vi "Dashboard Main.vi"() -> ()   [LabVIEW 2013]
uses:
  Vision Stuff/TargetType.ctl
  <vilib>/event_ctls.llb/eventvkey.ctl
  <vilib>/Rock Robotics/WPI/Dashboard/WPI_DashboardLogging Global.vi
  <vilib>/Utility/config.llb/Write Key (String).vi
  <vilib>/Utility/config.llb/Write Key (I32).vi
  <vilib>/Utility/config.llb/NI_LVConfig.lvlib
panel:
  out "Image Message":string="Timeout in Camera Communications"
  in  "Rec Mode":enum32{"Stop", "Record", "Playback"}(radio)
  in  "Dashboard Tab":T1(tab)
  in  "PID rotation":bool
  in  "Use Gyro":bool=TRUE
  in  "Camera Settings":T2={"Frame Rate"=30, "Compression"=30, "Size"=1} {"Frame Rate" scale=1.0..30.0; "Size" items=["640x480", "320x240", "160x120"]}
  out "MotorSliders R":cluster{"MotorSlide1":dbl, "MotorSlide2":dbl} {"MotorSlide2" scale=-1.0..1.0 scale format="%#_2e"; "MotorSlide1" scale=-1.0..1.0 scale format="%#_2e"}
  out "MotorChart R":cluster{"Numeric":dbl, "Numeric":dbl}(graph)
  out "MotorSliders L":T3 {"MotorSlide4 2" scale=0.0..14.0 scale format="%#_2e"; "MotorSlide2" scale=-1.0..1.0 scale format="%#_2e"; "MotorSlide1" scale=-1.0..1.0 scale format="%#_2e"}
  out "MotorChart L":T4(graph)
  out "JS1 Z":dbl(slide) scale=-1.0..1.0 scale format="%#_2e"
  out "Joystick 1":cluster{"X":dbl, "Y":dbl}[](graph)
  out "JS Buttons 1":T5
  out "JS2 Z":dbl(slide) scale=-1.0..1.0 scale format="%#_2e"
  out "Joystick 2":cluster{"X":dbl, "Y":dbl}[](graph)
  out "JS Buttons 2":T5
  out "Mode":T6(ring)=enum."Auto Disabled"
  out "Camera IP":string
  in  "DB Camera Config":bool
  out "fps":dbl format="%#.1g"
  out "Mbps":dbl format="%#.1g"
  out "Mbps 2":bool
  out "LED 1":bool
  in  "Op joystick select":string(combo)="Regular"
  in  "Driver joystick select":string(combo)="Regular"
  in  "Automatic reload?":bool
  out "Ultrasonic":dbl
  in  "Joystick":dbl=4.2
  in  "Gain":dbl=0.03
  out "Angle":dbl(knob) scale=0.0..360.0
  out "Hardstop position":bool
  out "Hardstop RPM":dbl
  out "Hardstop Encoder Distance":dbl
  in  "Slider 1":dbl(slide) scale=0.0..100.0
  in  "Value":dbl
  in  "Var#":dbl
  in  "Auton#":dbl
  in  "Update":bool
  in  "Auton's":string(combo)="OneBall"
  in  "Checkbox 2":bool
  in  "Checkbox 1":bool
  in  "Test Slider":dbl(slide) scale=0.0..100.0 scale format="%#_3g"
  in  "On/Off":bool caption="Solenoid"
  in  "Test Name":u16(ring) items=["Select the test to run...", "Example Test", "-------------------------------", "List of tests is built in robot code.", "Replace with your own automated tests."]
  in  "Test Tree":string(tree)
  in  "Motor":cluster{"Value":dbl, "Enable":bool} {"Value" scale=-1.0..1.0 scale format="%#_3g"}
  out "Progress":T7 {"Test Progress" scale=0.0..100.0}
  in  "Rev/Fwd":cluster{"Forward":bool, "Reverse":bool}
  in  "Test Ring":u16(ring) items=["Auto", "Fixed indoor", "Fixed outdoor 1", "Fixed outdoor 2", "Fixed fluorescent 1", "Fixed fluorescent 2", "Hold current"]
  in  "Listbox":i32(listbox)
  out "Tree":string(tree)
  out "Scores.State":T8
  out "Distance (ft)":dbl
  out "Heatmap":T9(plugin-control)
  out "Camera Image 2":T9(plugin-control)
  out "Ball X-Axis":sgl
  out "Camera Image":T9(plugin-control)
  in  "Enable":bool=TRUE
  # "ON"
  # "ON"
  # "OFF"
  # "Left"
  # "Front"
  # "Right"
  # "OFF"
  # "ON"
  # "Battery"
  # "OFF"
  # "Customize by placing controls and indicators here and name to\nmatch Dashboard Variables on robot."
  # "This tab is a great place for autonomous settings and validation.\nCustomize by placing controls and indicators here and name to\nmatch Dashboard Variables on robot."
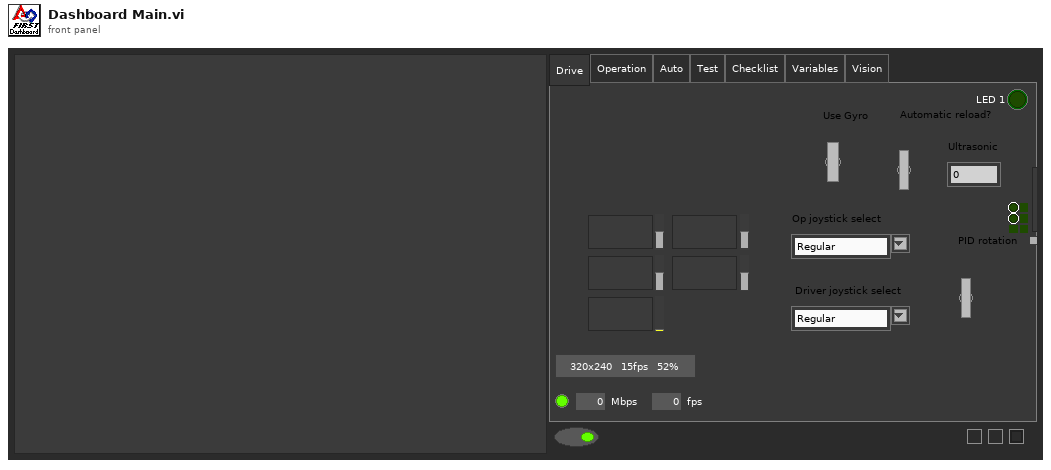
[diagram p1: front panel]
types:
  T1 = enum32{"Drive", "Operation", "Auto", "Test", "Checklist", "Variables", "Vision"}
  T2 = cluster{"Frame Rate":i32, "Compression":i32, "Size":u16}
  T3 = cluster{"MotorSlide1":dbl, "MotorSlide2":dbl, "MotorSlide4 2":dbl}
  T4 = cluster{"Numeric":dbl, "Numeric":dbl, "Battery":sgl}
  T5 = cluster{bool, bool, bool, bool, bool, bool, bool, bool, bool, bool, bool, bool}
  T6 = enum8{"Tele-Op Disabled", "Tele-Op Enabled", "Auto Disabled", "Auto Enabled", "Test Disabled", "Test Enabled", ""}
  T7 = cluster{"Test Progress":u8, "Test Progress Text":string}
  T8 = typedef "TargetType.ctl" = enum16{"Not Hot", "Hot"}
  T9 = typedef "IMAQ Image.ctl" = refnum<image>
  T10 = typedef "Image Type" = u32
  T11 = enum32{"Drive", "Operation", "Auto", "Test", "Checklist", "Variables"}
  T12 = cluster{"Score":sgl, "Fitted Circle":cluster{"Center":cluster{"X":sgl, "Y":sgl}, "Radius":dbl, "Circle Rect":cluster{"L":sgl, "T":sgl, "R":sgl, "B":sgl}, "Roundness":dbl, "SNR (dB)":dbl}, "Search Rect":cluster{"L":sgl, "T":sgl, "R":sgl, "B":sgl}, "Details":cluster{"Edge":sgl, "Area":sgl, "Circ":sgl, "Diam":sgl}}[]
  T13 = cluster{"Score":sgl, "Fitted Circle":cluster{"Center":cluster{"X":sgl, "Y":sgl}, "Radius":dbl, "Circle Rect":cluster{"L":sgl, "T":sgl, "R":sgl, "B":sgl}, "Roundness":dbl, "SNR (dB)":dbl}, "Search Rect":cluster{"L":sgl, "T":sgl, "R":sgl, "B":sgl}, "Details":cluster{"Edge":sgl, "Area":sgl, "Circ":sgl, "Diam":sgl}}
  T14 = cluster{"Scores":cluster{"Total":dbl, "Left":dbl, "Right":dbl, "Ratio":dbl, "Vertical":dbl, "index":i32, "State":T8}, "Verticals":cluster{"Horizontal?":bool, "Aspect Score":dbl, "Rect Score":dbl, cluster{"Left":dbl, "Top":dbl, "Right":dbl, "Bottom":dbl}, "Equiv H":dbl, "Equiv V":dbl}, "Horizontals":cluster{"Horizontal?":bool, "Aspect Score":dbl, "Rect Score":dbl, cluster{"Left":dbl, "Top":dbl, "Right":dbl, "Bottom":dbl}, "Equiv H":dbl, "Equiv V":dbl}, "Distance ft":dbl, "Center":cluster{"X":dbl, "Y":dbl}}[]
  T15 = cluster{"Scores":cluster{"Total":dbl, "Left":dbl, "Right":dbl, "Ratio":dbl, "Vertical":dbl, "index":i32, "State":T8}, "Verticals":cluster{"Horizontal?":bool, "Aspect Score":dbl, "Rect Score":dbl, cluster{"Left":dbl, "Top":dbl, "Right":dbl, "Bottom":dbl}, "Equiv H":dbl, "Equiv V":dbl}, "Horizontals":cluster{"Horizontal?":bool, "Aspect Score":dbl, "Rect Score":dbl, cluster{"Left":dbl, "Top":dbl, "Right":dbl, "Bottom":dbl}, "Equiv H":dbl, "Equiv V":dbl}, "Distance ft":dbl, "Center":cluster{"X":dbl, "Y":dbl}}
  T16 = typedef "NI_LVConfig.lvlib/Config Data RefNum.ctl" = refnum<k1>
  T17 = cluster{"Digital Inputs":bool[], "Digital Outputs":bool[]}
  T18 = cluster{"Competition mode":bool, "Robot Link":bool, "Autonomous":bool, "Enabled":bool, "E-Stop":bool, "Simulated":bool, "TestMode":bool, "Docked Window":bool}
  T19 = cluster{"Boolean Array[0]":bool, "Boolean Array[1]":bool, "Boolean Array[2]":bool, "Boolean Array[3]":bool, "Boolean Array[4]":bool, "Boolean Array[5]":bool, "Boolean Array[6]":bool, "Boolean Array[7]":bool, "Boolean Array[8]":bool, "Boolean Array[9]":bool, "Boolean Array[10]":bool, "Boolean Array[11]":bool}
  T20 = typedef "eventvkey.ctl" = enum16{"ASCII", "Enter", "Return", "Shift", "Ctrl", "Alt", "Cmd", "Opt", "Caps", "NumLock", "Clear", "Break", "Up", "Down", "Left", "Right", "Insert", "Delete", "Home", "End", "PageUp", "PageDown", "Escape", "Help", "Pause", "ScrollLock", "F1", "F2", "F3", "F4", "F5", "F6", "F7", "F8", "F9", "F10", "F11", "F12", "F13", "F14", "F15", "F16", "F17", "F18", "F19", "F20", "F21", "F22", "F23", "F24", "Play", "VolumeUp", "VolumeDown", "Mute", "Two Byte Char"}
  T21 = cluster{"Image Size":bool, "Image Type":bool, "Pixel Value":bool, "ROI Information":bool, "Zoom Factor":bool}
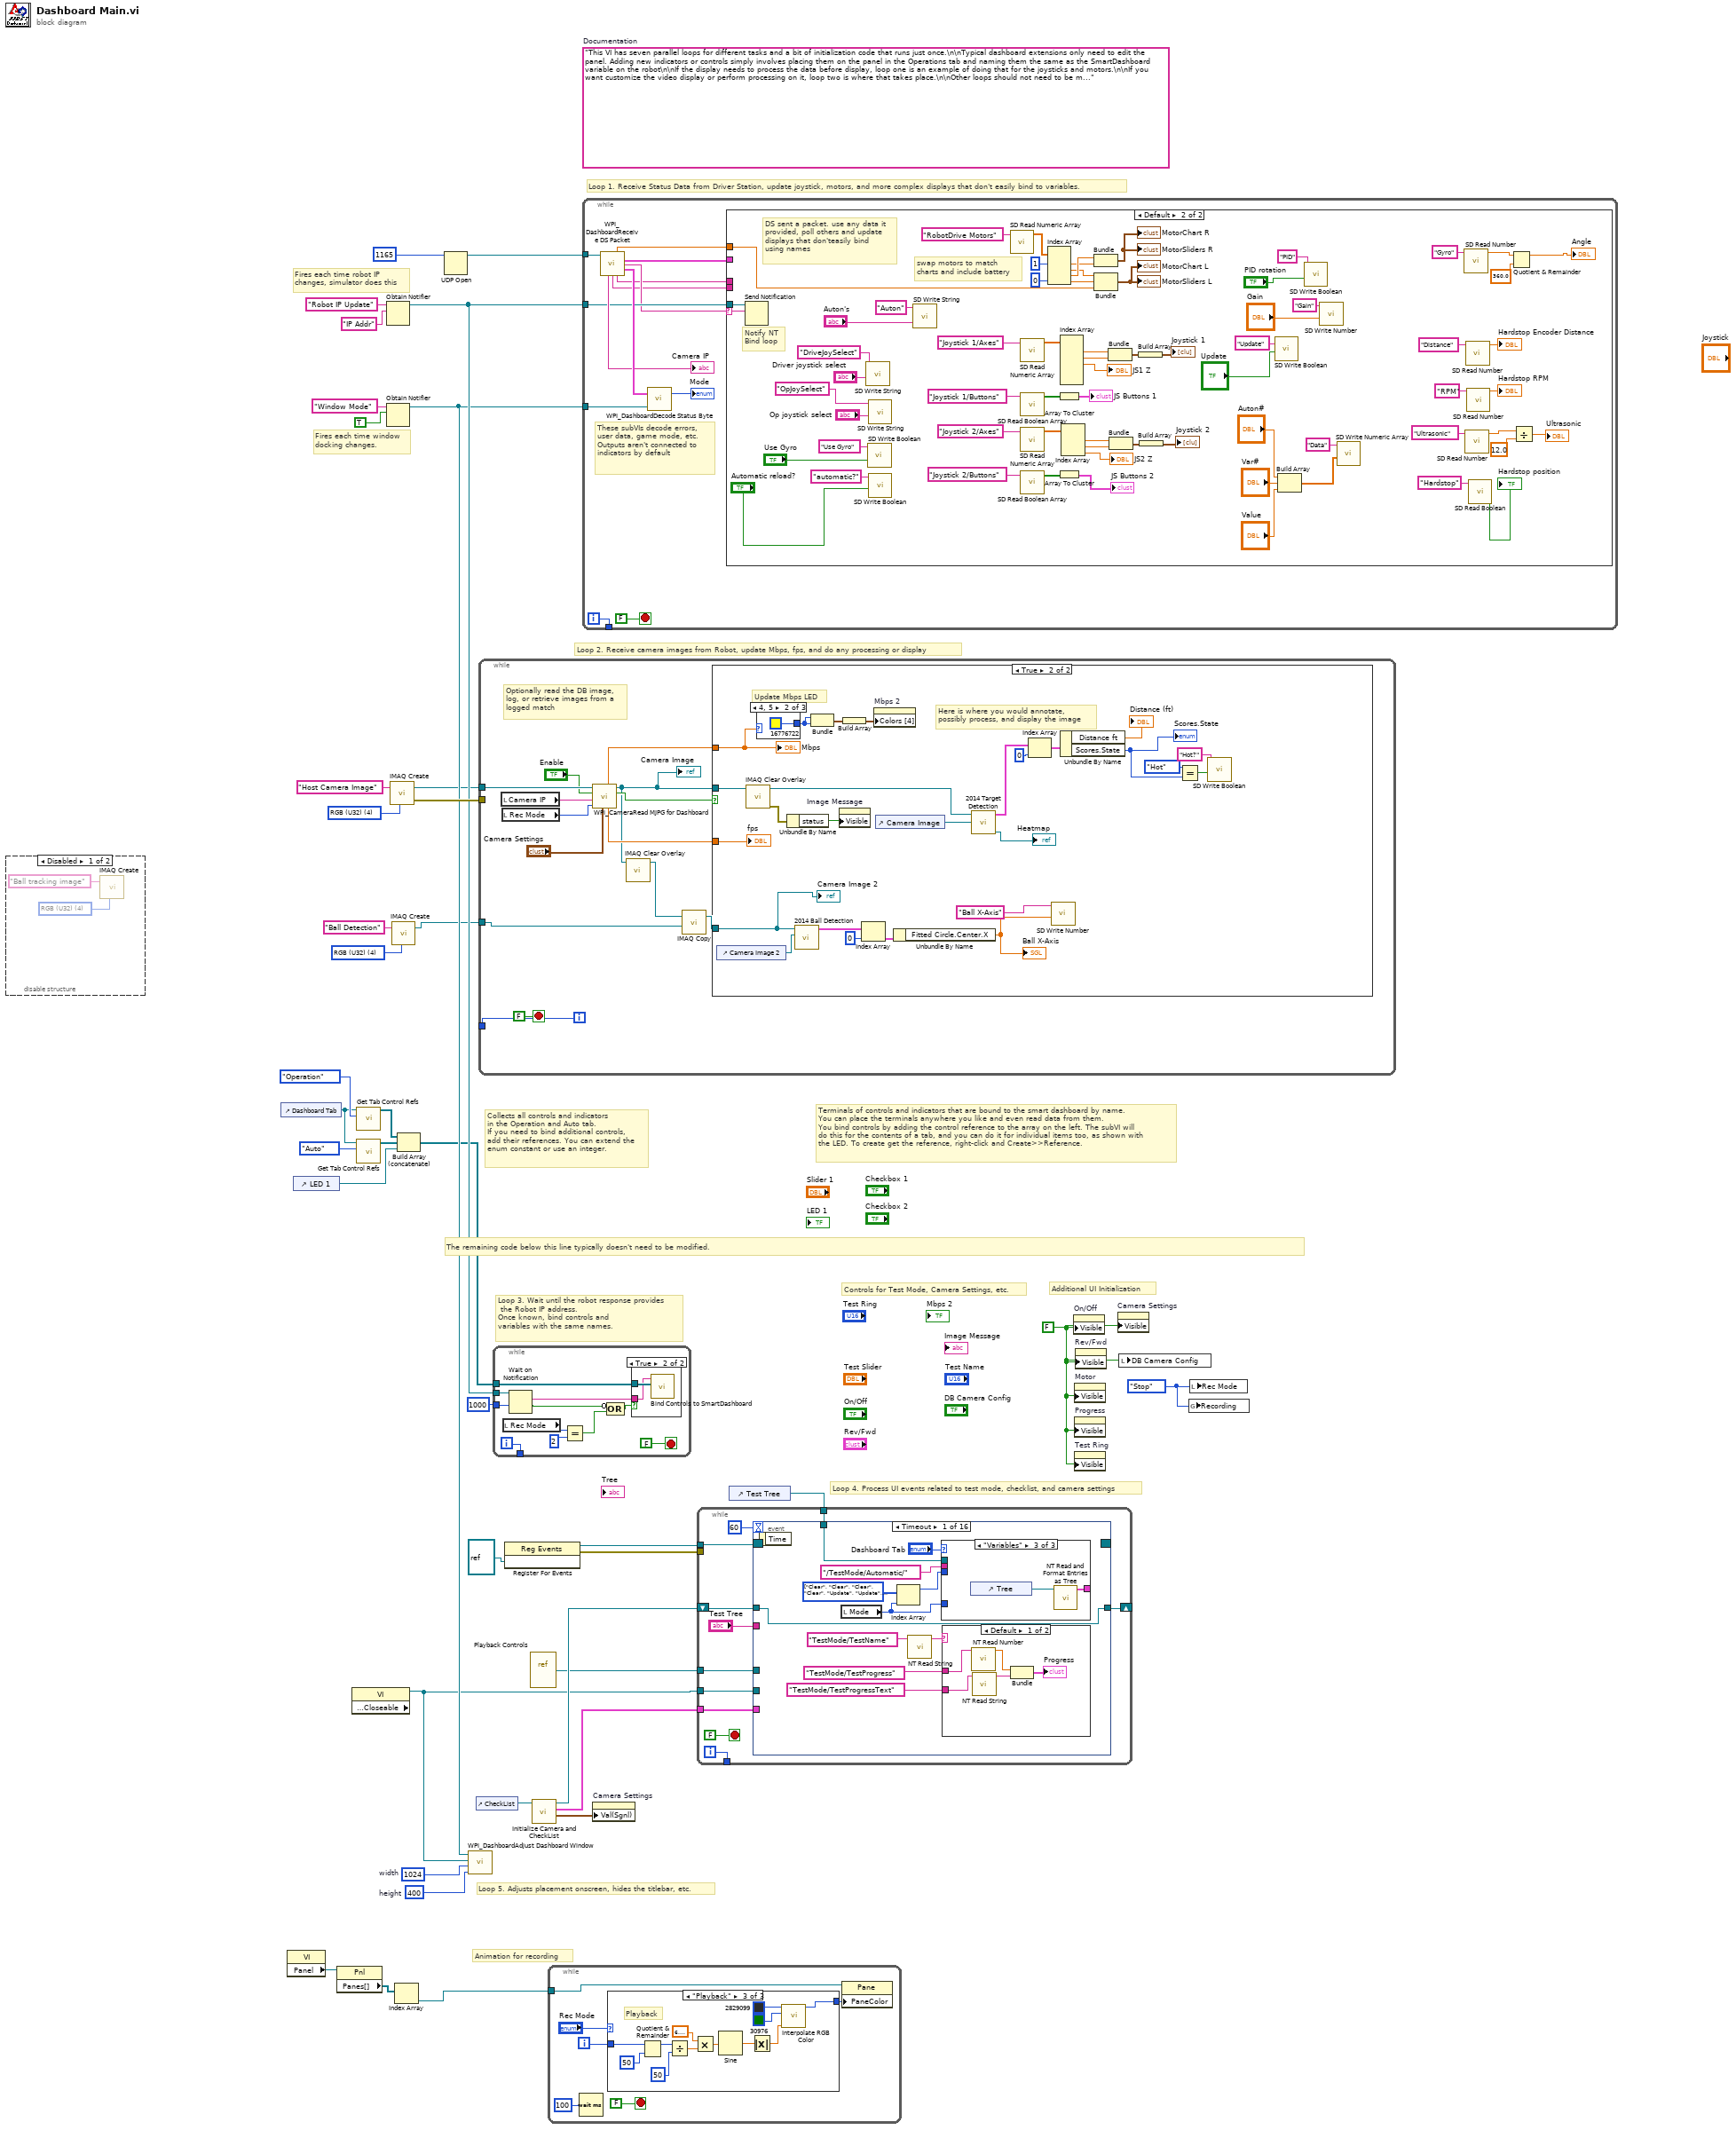
[diagram p0: block diagram]
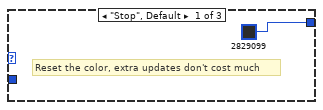
[diagram p3: hidden frame]
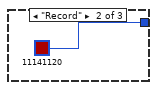
[diagram p4: hidden frame]
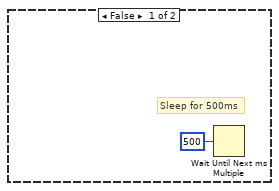
[diagram p6: hidden frame]
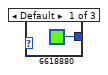
[diagram p7: hidden frame]
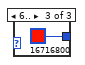
[diagram p8: hidden frame]
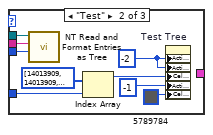
[diagram p10: hidden frame]
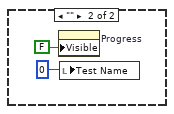
[diagram p11: hidden frame]
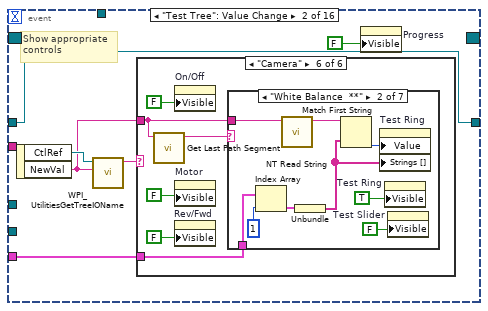
[diagram p12: hidden frame]
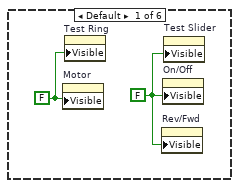
[diagram p13: hidden frame]
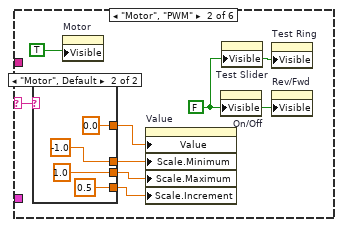
[diagram p14: hidden frame]
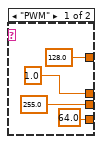
[diagram p15: hidden frame]
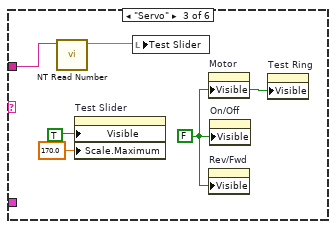
[diagram p16: hidden frame]
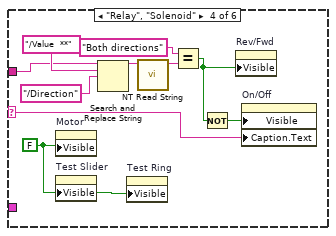
[diagram p17: hidden frame]
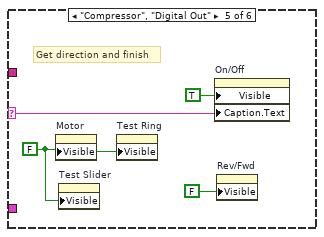
[diagram p18: hidden frame]
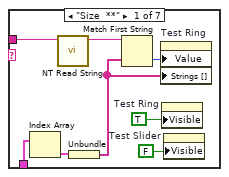
[diagram p19: hidden frame]
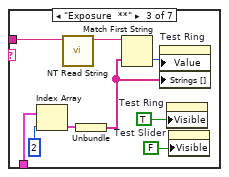
[diagram p20: hidden frame]
diagram:
  w2 = T10 4 items=["Grayscale (U8)", "Grayscale (I16)", "Grayscale (SGL)", "Complex (CSG)", "RGB (U32)", "HSL (U32)", "RGB (U64)", "Grayscale (U16)"] ("Image Type")
  w12 = enum32{"Stop", "Record", "Playback"}."Stop" ("Rec Mode")
  w15 = 400  # height
  w16 = 1024  # width
  w29 = FALSE ("Visible")
  (unwired) "This VI has seven parallel loops for different tasks and a bit of initialization code that runs just once.\n\nTypical dashboard extensions only need to edit the panel. Adding new indicators or controls simply involves placing them on the panel in the Operations tab and naming them the same as the SmartDashboard variable on the robot\n\nIf the display needs to process the data before display, loop one is an example of doing that for the joysticks and motors.\n\nIf you want customize the video display or perform processing on it, loop two is where that takes place.\n\nOther loops should not need to be modified. They are pretty standard, and document the task they perform."  # Documentation
  w38 = T10 4 items=["Grayscale (U8)", "Grayscale (I16)", "Grayscale (SGL)", "Complex (CSG)", "RGB (U32)", "HSL (U32)", "RGB (U64)"] ("Image Type")
  # "Controls for Test Mode, Camera Settings, etc."
  # "Additional UI Initialization"
  # "Animation for recording"
  # "Fires each time robot IP\nchanges, simulator does this"
  # "Fires each time window\ndocking changes."
  # "Collects all controls and indicators\nin the Operation and Auto tab.\nIf you need to bind additional controls,\nadd their references. You can extend the\nenum constant or use an integer."
  # "The remaining code below this line typically doesn't need to be modified."
  # "Loop 4. Process UI events related to test mode, checklist, and camera settings"
  # "Terminals of controls and indicators that are bound to the smart dashboard by name.\nYou can place the terminals anywhere you like and even read data from them.\nYou bind controls by adding the control reference to the array on the left. The subVI will\ndo this for the contents of a tab, and you can do it for individual items too, as shown with\nthe LED. To create get the reference, right-click and Create>>Reference."
  # "Loop 3. Wait until the robot response provides\n the Robot IP address.\nOnce known, bind controls and\nvariables with the same names."
  # "Loop 5. Adjusts placement onscreen, hides the titlebar, etc."
  # "Loop 1. Receive Status Data from Driver Station, update joystick, motors, and more complex displays that don't easily bind to variables."
  # "Loop 2. Receive camera images from Robot, update Mbps, fps, and do any processing or display"
  n1 = disable-structure shown="Disabled" {
    frame Disabled {
      w41 = T10 4 items=["Grayscale (U8)", "Grayscale (I16)", "Grayscale (SGL)", "Complex (CSG)", "RGB (U32)", "HSL (U32)", "RGB (U64)"] ("Image Type")
      n2 = call "IMAQ Create"("Image Name"="Ball tracking image", "Image Type"=w41) -> ()  [unwired: 2 in, 3 out]
    }
    frame Enabled {
    }
  }
  n3 = control-ref of="Dashboard Tab"() -> (w10:refnum<vi>)
  n4 = property class="VI"() -> ("Panel"=w23:refnum<vi>)  [unwired: 2 in, 2 out]
  n5 = control-ref of="LED 1"() -> (w5:refnum<vi>)
  n6 = property class="Pnl"(reference=w23) -> ("Panes[]"=w24:refnum<vi>[])  [unwired: 1 in, 2 out]
  n7 = property class="VI" props=["Front Panel.Closeable"]() -> (reference out=w11:refnum<vi>)  [unwired: 2 in, 2 out]
  n8 = call <vilib>:"Get Tab Control Refs.vi"("Page Index"=T11."Operation" ("Dashboard Tab"), "TabControl in"=w10) -> ("ControlsOnPage"=w8:refnum<vi>[])  [unwired: 9 in]
  n9 = call <vilib>:"Get Tab Control Refs.vi"("Page Index"=T11."Auto" ("Dashboard Tab"), "TabControl in"=w10) -> ("ControlsOnPage"=w9:refnum<vi>[])  [unwired: 9 in]
  n10 = Obtain Notifier(name (unnamed)="Robot IP Update", notification data type="IP Addr" ("name (unnamed)")) -> (notifier out=w33:refnum<notifier>)  [unwired: 2 in, 2 out]
  n11 = Obtain Notifier(name (unnamed)="Window Mode", notification data type=TRUE) -> (notifier out=w14:refnum<notifier>)  [unwired: 2 in, 2 out]
  n12 = call "IMAQ Create"("Image Name"="Host Camera Image", "Image Type"=w38) -> ("New Image"=w4:T9, "error out"=w36:errorcluster)  [unwired: 2 in, 1 out]
  n13 = call "IMAQ Create"("Image Name"="Ball Detection", "Image Type"=w2) -> ("New Image"=w1:T9)  [unwired: 2 in, 2 out]
  n14 = Index Array(array=w24) -> (element=w22:refnum<vi>)  [unwired: 1 in]
  n15 = Build Array (concatenate)(w8, w9, w5) -> (w7:refnum<vi>[])
  n16 = UDP Open(11:u16 1165 ("port")) -> (port=w39:refnum<k16>)  [unwired: 2 in, 4 out]
  n17 = call <vilib>:"WPI_DashboardAdjust Dashboard Window.vi"("height"=w15, "width"=w16, "reference in"=w11, "Notifier in"=w14) -> ()  [unwired: 8 in]
  n18 = control-ref of="CheckList"() -> (w13:refnum<vi>)
  n19 = while {
    tunnel: w4 -> [w54]
    tunnel: w36 -> [_]
    tunnel: [w55] -> _
    tunnel: w1 -> [w46]
    i -> [w55]
    stop <- FALSE stop-if-true
    # "Optionally read the DB image,\nlog, or retrieve images from a\nlogged match"
    n20 = local read "Camera IP"() -> (w49:string)
    n21 = local read "Rec Mode"() -> (w50:enum32{"Stop", "Record", "Playback"})
    n22 = call <vilib>:"WPI_CameraRead MJPG for Dashboard.vi"("Camera Settings"="Camera Settings", "Rec Mode"=w50, "Camera IP"=w49, "Enable"="Enable", "Refnum in"=w54) -> ("Active"=w53:bool, "Refnum out"=w45:T9, "FPS"=w52:dbl, "Bandwidth (Mbps)"=w51:dbl)  [unwired: 3 in]
    "Camera Image" <- w45
    n23 = call "IMAQ Clear Overlay"("Image"=w45) -> ("Image Out"=w44:T9)  [unwired: 2 in, 8 out]
    n24 = call "IMAQ Copy"("Image Dst"=w46, "Image Src"=w44) -> ("Image Dst Out"=w43:T9)  [unwired: 4 in, 1 out]
    n25 = case shown="True" w53 {
      tunnel: w45 -> [_ w66]
      tunnel: w51 -> [_ w78]
      tunnel: w52 -> [_ w67]
      tunnel: w43 -> [_ w59]
      frame False {
        # "Sleep for 500ms"
        n26 = Wait Until Next ms Multiple(millisecond multiple=u32 500) -> ()  [unwired: 1 out]
      }
      frame True {
        # "Here is where you would annotate,\npossibly process, and display the image"
        # "Update Mbps LED"
        n27 = control-ref of="Camera Image 2"() -> (w58:refnum<vi>)
        n28 = call "IMAQ Clear Overlay"("Image"=w66) -> ("error out"=w82:errorcluster, "Image Out"=w65:T9)  [unwired: 2 in, 7 out]
        n29 = case shown="4, 5" w78 {
          tunnel: [u32 6618880 ("Color Box") u32 16776722 ("Color Box") u32 16716800 ("Color Box")] -> w79
          frame Default {
          }
          frame 4, 5 {
          }
          frame 6.. {
          }
        }
        n30 = Unbundle By Name(w82) -> ("status"=w83:bool)
        n31 = call "2014 Ball Detection.vi"("Image Ctl Refnum"=w58, "Src Image"=w59) -> ("Ranked Objects"=w64:T12)  [unwired: 8 in, 1 out]
        n32 = Bundle("Color Box"=w79, "Color Box"=w79) -> (w81:cluster{"Color Box":u32, "Color Box":u32})  [unwired: 1 out]
        n33 = property on="Image Message" class="Str"("Visible"=w83) -> ()  [unwired: 2 in, 2 out]
        n34 = Build Array(w81) -> (w80:cluster{"Color Box":u32, "Color Box":u32}[])
        n35 = Index Array(array=w64, index=0) -> (element=w62:T13)
        n36 = property on="Mbps 2" class="Bool (strict)"("Colors [4]"=w80) -> ()  [unwired: 2 in, 2 out]
        n37 = control-ref of="Camera Image"() -> (w77:refnum<vi>)
        n38 = Unbundle By Name(w62) -> ("Fitted Circle.Center.X"=w60:sgl)
        "Ball X-Axis" <- w60
        n39 = call "2014 Target Detection.vi"("Image Ctl Refnum"=w77, "Image in"=w65) -> ("Mask"=→"Heatmap":T9, "Target Info"=w76:T14)  [unwired: 7 in, 1 out]
        n40 = Index Array(array=w76, index=0) -> (element=w74:T15)
        n41 = call <vilib>:"SD Write Number.vi"("Numeric"=w60, "Name"="Ball X-Axis") -> ()  [unwired: 8 in, 2 out]
        n42 = Unbundle By Name(w74) -> ("Distance ft"=→"Distance (ft)":dbl, "Scores.State"=w72:T8)
        "Scores.State" <- w72
        n43 = Equal?(x=TargetType."Hot", y=w72) -> (x = y?=w70:bool)
        n44 = call <vilib>:"SD Write Boolean.vi"("Boolean"=w70, "Name"="Hot?") -> ()  [unwired: 8 in, 2 out]
        "Mbps" <- w78
        "fps" <- w67
        "Camera Image 2" <- w59
      }
    }
  }
  n45 = while {
    tunnel: w7 -> [w97]
    tunnel: w33 -> [w95]
    tunnel: [w93] -> _
    tunnel: u32 1000 ("milliseconds to wait") -> [w92]
    i -> [w93]
    stop <- FALSE stop-if-true
    n46 = local read "Rec Mode"() -> (w88:enum32{"Stop", "Record", "Playback"})
    n47 = Wait on Notification(notifier=w95, timeout in ms (-1)=w92) -> (notification=w94:string, timed out?=w90:bool)  [unwired: 2 in, 2 out]
    n48 = Equal?(x=w88, y=u16 2 ("Rec Mode")) -> (x = y?=w89:bool)
    n49 = Compound Arithmetic op=OR(invert w90, w89) -> (w91:bool)
    n50 = case shown="True" w91 {
      tunnel: w97 -> [_ w99]
      tunnel: w94 -> [_ w98]
      frame False {
      }
      frame True {
        n51 = call <vilib>:"Bind Controls to SmartDashboard.vi"("Bound Control Refs"=w99, "Server IP Address"=w98) -> ()  [unwired: 10 in]
      }
    }
  }
  n52 = register-events(refnum<vi> refnum) -> (reference out=w20:refnum<event-registration>, error out=w19:errorcluster)  [unwired: 2 in]
  n53 = vi-ref "Playback Controls.vi"() -> (w21:refnum<vi>)
  n54 = call "Initialize Camera and CheckList.vi"("ListBox in"=w13) -> ("Cluster"=w27:cluster{"value":i32, "value":i32, "index":i32}, "Array"=w28:cluster{string[]}[], "File Refnum"=w26:T16)  [unwired: 8 in]
  n55 = while {
    tunnel: w22 -> [w101]
    i -> [w104]
    stop <- FALSE stop-if-true
    n56 = Wait (ms)(milliseconds to wait=u32 100) -> ()  [unwired: 1 out]
    n57 = case shown="\"Playback\"" "Rec Mode" {
      tunnel: w104 -> [_ _ w119]
      tunnel: [u32 2829099 ("Base Color") u32 11141120 ("Target Color") w108] -> w100
      frame "Stop", Default {
        # "Reset the color, extra updates don't cost much"
      }
      frame "Record" {
      }
      frame "Playback" {
        # "Playback"
        n58 = Quotient & Remainder(x=w119, y=u32 50 ("milliseconds to wait")) -> (x-y*floor(x/y)=w115:u32)  [unwired: 1 out]
        n59 = Divide(x=w115, y=u32 50 ("milliseconds to wait")) -> (x/y=w112:dbl)
        n60 = Multiply(x=6.283185307179586, y=w112) -> (x*y=w117:dbl)
        n61 = Sine(x=w117) -> (sin(x)=w116:dbl)
        n62 = Absolute Value(x=w116) -> (abs(x)=w109:dbl)
        n63 = call "Interpolate RGB Color.vi"("Proportion"=w109, "Target Color"=u32 30976, "Base Color"=u32 2829099) -> ("Result Color"=w108:u32)  [unwired: 8 in]
      }
    }
    n64 = property class="Pane"(reference=w101, "PaneColor"=w100) -> ()  [unwired: 1 in, 2 out]
  }
  n65 = while {
    tunnel: w39 -> [w130]
    tunnel: w33 -> [w125]
    tunnel: w14 -> [w129]
    tunnel: [w126] -> _
    i -> [w126]
    stop <- FALSE stop-if-true
    # "These subVIs decode errors, user data, game mode, etc.\nOutputs aren't connected to indicators by default"
    n66 = call <vilib>:"WPI_DashboardReceive DS Packet.vi"("Recv Socket"=w130) -> ("Battery"=w120:sgl, "Driver Station"=w121:T17, "Robot IP Address"=w124:string, "Status"=w131:T18, "Camera IP Address"=→"Camera IP":string, "Low Priority User Data"=w123:string, "High Priority User Data"=w122:string)  [unwired: 1 in, 7 out]
    n67 = call <vilib>:"WPI_DashboardDecode Status Byte.vi"("Window Mode Notifier"=w129, "Status"=w131) -> ("Mode"=→"Mode":T6)  [unwired: 1 out]
    n68 = case shown="Default" w124 {
      selector: w124 -> [_ w179]
      tunnel: w125 -> [_ w180]
      tunnel: w123 -> [_ _]
      tunnel: w122 -> [_ _]
      tunnel: w121 -> [_ _]
      tunnel: w120 -> [_ w178]
      frame "0.0.0.0" {
        # "DS not sending packets, or no robot exists yet.\nDon't poll the variables"
      }
      frame Default {
        # "Notify NT\nBind loop"
        # "DS sent a packet. use any data it\nprovided, poll others and update\ndisplays that don'teasily bind\nusing names"
        # "swap motors to match\ncharts and include battery"
        n69 = Send Notification(notification=w179, notifier=w180) -> ()  [unwired: 1 in, 2 out]
        n70 = call <vilib>:"SD Write String.vi"("String"="Driver joystick select", "Name"="DriveJoySelect") -> ()  [unwired: 8 in, 2 out]
        n71 = call <vilib>:"SD Write Boolean.vi"("Boolean"="Use Gyro", "Name"="Use Gyro") -> ()  [unwired: 8 in, 2 out]
        n72 = call <vilib>:"SD Write String.vi"("String"="Op joystick select", "Name"="OpJoySelect") -> ()  [unwired: 8 in, 2 out]
        n73 = call <vilib>:"SD Write Boolean.vi"("Boolean"="Automatic reload?", "Name"="automatic?") -> ()  [unwired: 8 in, 2 out]
        n74 = call <vilib>:"SD Write String.vi"("String"="Auton's", "Name"="Auton") -> ()  [unwired: 8 in, 2 out]
        n75 = call <vilib>:"SD Read Numeric Array.vi"("Name"="RobotDrive Motors") -> ("Numeric Array"=w177:dbl[])  [unwired: 8 in, 2 out]
        n76 = call <vilib>:"SD Read Numeric Array.vi"("Name"="Joystick 1/Axes") -> ("Numeric Array"=w195:dbl[])  [unwired: 8 in, 2 out]
        n77 = call <vilib>:"SD Read Boolean Array.vi"("Name"="Joystick 1/Buttons") -> ("Boolean Array"=w197:bool[])  [unwired: 8 in, 2 out]
        n78 = call <vilib>:"SD Read Numeric Array.vi"("Name"="Joystick 2/Axes") -> ("Numeric Array"=w189:dbl[])  [unwired: 8 in, 2 out]
        n79 = call <vilib>:"SD Read Boolean Array.vi"("Name"="Joystick 2/Buttons") -> ("Boolean Array"=w139:bool[])  [unwired: 8 in, 2 out]
        n80 = Index Array(array=w177, index #1=1, index #4=0) -> (element #1=w173:dbl, element #2=w172:dbl, element #3=w174:dbl, element #4=w169:dbl)  [unwired: 2 in]
        n81 = Array To Cluster(array=w197) -> (cluster=→"JS Buttons 1":T19)
        n82 = Array To Cluster(array=w139) -> (cluster=→"JS Buttons 2":T19)
        n83 = Index Array(array=w195) -> (element #1=w192:dbl, element #2=w193:dbl, element #3=→"JS1 Z":dbl)  [unwired: 6 in, 3 out]
        n84 = Index Array(array=w189) -> (element #1=w185:dbl, element #2=w184:dbl, element #3=→"JS2 Z":dbl)  [unwired: 3 in]
        n85 = Bundle("Numeric"=w174, "Numeric"=w173) -> (→"MotorChart R" →"MotorSliders R":cluster{"Numeric":dbl, "Numeric":dbl})  [unwired: 1 in]
        n86 = Bundle("Numeric"=w172, "Numeric"=w169, "Battery"=w178) -> (→"MotorChart L" →"MotorSliders L":T4)  [unwired: 1 in]
        n87 = Bundle("Numeric"=w192, "Numeric"=w193) -> (w191:cluster{"Numeric":dbl, "Numeric":dbl})  [unwired: 1 in]
        n88 = Bundle("Numeric"=w185, "Numeric"=w184) -> (w186:cluster{"Numeric":dbl, "Numeric":dbl})  [unwired: 1 in]
        n89 = Build Array(w191) -> (→"Joystick 1":cluster{"Numeric":dbl, "Numeric":dbl}[])
        n90 = Build Array(w186) -> (→"Joystick 2":cluster{"Numeric":dbl, "Numeric":dbl}[])
        n91 = call <vilib>:"SD Write Boolean.vi"("Boolean"="Update", "Name"="Update") -> ()  [unwired: 8 in, 2 out]
        n92 = Build Array("Auton#", "Var#", "Value") -> (w138:dbl[])
        n93 = call <vilib>:"SD Write Boolean.vi"("Boolean"="PID rotation", "Name"="PID") -> ()  [unwired: 8 in, 2 out]
        n94 = call <vilib>:"SD Write Number.vi"("Numeric"="Gain", "Name"="Gain") -> ()  [unwired: 8 in, 2 out]
        n95 = call <vilib>:"SD Write Numeric Array.vi"("Numeric Array"=w138, "Name"="Data") -> ()  [unwired: 8 in, 2 out]
        n96 = call <vilib>:"SD Read Number.vi"("Name"="Gyro") -> ("Numeric"=w147:dbl)  [unwired: 8 in, 2 out]
        n97 = call <vilib>:"SD Read Number.vi"("Name"="Ultrasonic") -> ("Numeric"=w150:dbl)  [unwired: 8 in, 2 out]
        n98 = call <vilib>:"SD Read Number.vi"("Name"="Distance") -> ("Numeric"=→"Hardstop Encoder Distance":dbl)  [unwired: 8 in, 2 out]
        n99 = call <vilib>:"SD Read Number.vi"("Name"="RPM") -> ("Numeric"=→"Hardstop RPM":dbl)  [unwired: 8 in, 2 out]
        n100 = call <vilib>:"SD Read Boolean.vi"("Name"="Hardstop") -> ("Boolean"=→"Hardstop position":bool)  [unwired: 8 in, 2 out]
        n101 = Quotient & Remainder(x=w147, y=360.0) -> (x-y*floor(x/y)=→"Angle":dbl)  [unwired: 1 out]
        n102 = Divide(x=w150, y=12.0) -> (x/y=→"Ultrasonic":dbl)
      }
    }
  }
  n103 = property on="Camera Settings" class="Clust (strict)"("Val(Sgnl)"=w27) -> ()  [unwired: 2 in, 2 out]
  n104 = control-ref of="Test Tree"() -> (w25:refnum<vi>)
  n105 = while {
    tunnel: w28 -> [w208]
    shift-right: [w207] -> _
    shift-left: w26 -> [w206]
    tunnel: [w205] -> _
    tunnel: w25 -> [w204]
    tunnel: w21 -> [w203]
    tunnel: w20 -> [w202]
    tunnel: w19 -> [_]
    tunnel: w11 -> [w201]
    i -> [w205]
    stop <- FALSE stop-if-true
    n106 = event shown="[0] Timeout" {
      selector: w202 -> [_ _ _ _ _ _ _ _ _ _ _ _ _ _ _ _]
      dyn-events: [_ _ _ _ _ _ _ _ _ _ _ _ _ w446 _ _] -> _
      timeout: u32 60 ("milliseconds to wait") -> [_ _ _ _ _ _ _ _ _ _ _ _ _ _ _ _]
      tunnel: w204 -> [w218 _ _ _ _ _ _ _ _ _ _ _ _ _ _ _]
      tunnel: "Test Tree" -> [_ _ _ _ _ _ _ _ w415 w423 w425 w429 w437 _ _ _]
      tunnel: w208 -> [_ w242 _ _ _ _ w379 w409 _ _ _ _ _ _ _ _]
      tunnel: [w212 w241 w340 w345 w353 w365 w378 w402 w414 w421 w424 w428 w436 w448 w462 w463] -> w207
      tunnel: w206 -> [w212 w241 w340 w345 w353 w365 w377 w402 w414 w421 w424 w428 w436 w448 w462 w463]
      tunnel: w203 -> [_ _ _ _ _ _ _ _ _ _ _ _ _ w449 _ w466]
      tunnel: w201 -> [_ _ _ _ _ _ _ _ _ _ _ _ _ w444 _ _]
      event Timeout {
        w217 = enum16{"Update", "Clear"}[] [enum."Clear", enum."Clear", enum."Clear", enum."Clear", enum."Update", enum."Update", enum."Clear"] items=["Update", "Clear"]
        n107 = event-data() -> ()  [unwired: 1 in, 1 out]
        n108 = local read "Mode"() -> (w215:T6)
        n109 = Index Array(array=w217, index=w215) -> (element=w216:enum16{"Update", "Clear"})
        n110 = call <vilib>:"NT Read String.vi"("Name"="TestMode/TestName") -> ("String"=w221:string)  [unwired: 9 in, 1 out]
        n111 = case shown="\"Variables\"" "Dashboard Tab" {
          tunnel: w218 -> [_ w231 _]
          tunnel: "/TestMode/Automatic/" ("Name Pattern") -> [_ w230 _]
          tunnel: w216 -> [_ w229 _]
          tunnel: w215 -> [_ w227 _]
          tunnel: [_ _ w233] -> _
          frame "Operation", Default {
          }
          frame "Test" {
            w226 = -2 ("Active Item:Row Number")
            n112 = call <vilib>:"NT Read and Format Entries as Tree.vi"("Operation"=w229, "Name Pattern"=w230, "Tree Refnum"=w231) -> ()  [unwired: 7 in, 2 out]
            n113 = Index Array(array=u32[] [14013909, 14013909, 14013909, 14013909, 14013909, 16777215, 14013909], index=w227) -> (element=w225:u32)
            n114 = property on="Test Tree" class="Tree (strict)"("Active Item Row Number"=w226, "ActiveColNum"=w226, "CellBG"=w225, "Active Item Row Number"=-1 ("Active Item:Row Number"), "CellBG"=u32 5789784 ("Color Box")) -> ()  [unwired: 2 in, 2 out]
          }
          frame "Variables" {
            n115 = control-ref of="Tree"() -> (w232:refnum<vi>)
            n116 = call <vilib>:"NT Read and Format Entries as Tree.vi"("Tree Refnum"=w232) -> ("Formatted Strings"=w233:cluster{"Name":string, "Value":string}[])  [unwired: 9 in, 1 out]
          }
        }
        n117 = case shown="Default" w221 {
          tunnel: "TestMode/TestProgress" ("Name") -> [w235 _]
          tunnel: "TestMode/TestProgressText" ("Name") -> [w234 _]
          frame Default {
            n118 = call <vilib>:"NT Read Number.vi"("Name"=w235) -> ("Numeric"=w236:dbl)  [unwired: 9 in, 1 out]
            n119 = call <vilib>:"NT Read String.vi"("Name"=w234) -> ("String"=w237:string)  [unwired: 9 in, 1 out]
            n120 = Bundle("Numeric"=w236, "String"=w237) -> (→"Progress":cluster{"Numeric":dbl, "String":string})  [unwired: 1 in]
          }
          frame "" {
            n121 = property on="Progress" class="Clust (strict)"("Visible"=FALSE) -> ()  [unwired: 2 in, 2 out]
            n122 = local write "Test Name"(u16 0) -> ()
          }
        }
      }
      event "Test Tree": Value Change {
        # "Show appropriate\ncontrols"
        n123 = event-data() -> ("CtlRef"=w245:refnum<vi>, "NewVal"=w243:string)  [unwired: 1 in]
        n124 = call <vilib>:"WPI_UtilitiesGetTreeIOName.vi"("NewVal"=w243, "TreeControl in"=w245) -> ("I/O Name"=w246:string)  [unwired: 9 in]
        n125 = case shown="\"Camera\"" w246 {
          selector: w246 -> [_ w253 _ w271 w280 _]
          tunnel: w243 -> [_ _ w268 w270 _ w287]
          tunnel: w242 -> [_ _ _ _ _ w286]
          frame Default {
            w248 = FALSE ("Visible")
            w247 = FALSE ("Visible")
            n126 = property on="Motor" class="Clust (strict)"("Visible"=w247) -> ()  [unwired: 2 in, 2 out]
            n127 = property on="Test Ring" class="Ring (strict)"("Visible"=w247) -> ()  [unwired: 2 in, 2 out]
            n128 = property on="Rev/Fwd" class="Clust (strict)"("Visible"=w248) -> ()  [unwired: 2 in, 2 out]
            n129 = property on="On/Off" class="Bool (strict)"("Visible"=w248) -> ()  [unwired: 2 in, 2 out]
            n130 = property on="Test Slider" class="Slide (strict)"("Visible"=w248) -> ()  [unwired: 2 in, 2 out]
          }
          frame "Motor", "PWM" {
            w254 = FALSE ("Visible")
            n131 = case shown="\"Motor\", Default" w253 {
              tunnel: [1.0 ("Value") -1.0 ("Value")] -> w252
              tunnel: [255.0 ("Value") 1.0 ("Value")] -> w251
              tunnel: [128.0 ("Value") 0.0 ("Value")] -> w250
              tunnel: [64.0 ("Value") 0.5 ("Value")] -> w249
              frame "PWM" {
              }
              frame "Motor", Default {
              }
            }
            n132 = property on="Motor" class="Clust (strict)"("Visible"=TRUE) -> ()  [unwired: 2 in, 2 out]
            n133 = property on="Value" class="Slide (strict)"("Value"=w250, "Scale.Minimum"=w252, "Scale.Maximum"=w251, "Scale.Increment"=w249) -> ()  [unwired: 2 in, 2 out]
            n134 = property on="On/Off" class="Bool (strict)"("Visible"=w254) -> ()  [unwired: 2 in, 2 out]
            n135 = property on="Test Slider" class="Slide (strict)"("Visible"=w254) -> ()  [unwired: 2 in, 2 out]
            n136 = property on="Test Ring" class="Ring (strict)"("Visible"=w254) -> ()  [unwired: 2 in, 2 out]
            n137 = property on="Rev/Fwd" class="Clust (strict)"("Visible"=w254) -> ()  [unwired: 2 in, 2 out]
          }
          frame "Servo" {
            w266 = FALSE ("Visible")
            n138 = call <vilib>:"NT Read Number.vi"("Name"=w268) -> ("Numeric"=w267:dbl)  [unwired: 9 in, 1 out]
            n139 = property on="Test Slider" class="Slide (strict)"("Visible"=TRUE, "Scale.Maximum"=170.0 ("Scale.Range:Maximum")) -> ()  [unwired: 2 in, 2 out]
            n140 = local write "Test Slider"(w267) -> ()
            n141 = property on="Motor" class="Clust (strict)"("Visible"=w266) -> ()  [unwired: 2 in, 2 out]
            n142 = property on="Rev/Fwd" class="Clust (strict)"("Visible"=w266) -> ()  [unwired: 2 in, 2 out]
            n143 = property on="On/Off" class="Bool (strict)"("Visible"=w266) -> ()  [unwired: 2 in, 2 out]
            n144 = property on="Test Ring" class="Ring (strict)"("Visible"=w266) -> ()  [unwired: 2 in, 2 out]
          }
          frame "Relay", "Solenoid" {
            w269 = FALSE ("Visible")
            n145 = property on="Motor" class="Clust (strict)"("Visible"=w269) -> ()  [unwired: 2 in, 2 out]
            n146 = property on="Test Slider" class="Slide (strict)"("Visible"=w269) -> ()  [unwired: 2 in, 2 out]
            n147 = Search and Replace String(input string=w270, search string="/Value  **", replace string="/Direction") -> (result string=w276:string)  [unwired: 5 in, 3 out]
            n148 = property on="Test Ring" class="Ring (strict)"("Visible"=w269) -> ()  [unwired: 2 in, 2 out]
            n149 = call <vilib>:"NT Read String.vi"("Name"=w276) -> ("String"=w274:string)  [unwired: 9 in, 1 out]
            n150 = Equal?(x="Both directions", y=w274) -> (x = y?=w272:bool)
            n151 = Not(x=w272) -> (.not. x?=w273:bool)
            n152 = property on="Rev/Fwd" class="Clust (strict)"("Visible"=w272) -> ()  [unwired: 2 in, 2 out]
            n153 = property on="On/Off" class="Bool (strict)"("Visible"=w273, "Caption.Text"=w271) -> ()  [unwired: 2 in, 2 out]
          }
          frame "Compressor", "Digital Out" {
            w279 = FALSE ("Visible")
            # "Get direction and finish"
            n154 = property on="Motor" class="Clust (strict)"("Visible"=w279) -> ()  [unwired: 2 in, 2 out]
            n155 = property on="Test Slider" class="Slide (strict)"("Visible"=w279) -> ()  [unwired: 2 in, 2 out]
            n156 = property on="Test Ring" class="Ring (strict)"("Visible"=w279) -> ()  [unwired: 2 in, 2 out]
            n157 = property on="On/Off" class="Bool (strict)"("Visible"=TRUE, "Caption.Text"=w280) -> ()  [unwired: 2 in, 2 out]
            n158 = property on="Rev/Fwd" class="Clust (strict)"("Visible"=FALSE) -> ()  [unwired: 2 in, 2 out]
          }
          frame "Camera" {
            n159 = call <vilib>:"Get Last Path Segment.vi"("String in"=w287) -> ("String out"=w288:string)  [unwired: 10 in]
            n160 = property on="On/Off" class="Bool (strict)"("Visible"=FALSE) -> ()  [unwired: 2 in, 2 out]
            n161 = property on="Motor" class="Clust (strict)"("Visible"=FALSE) -> ()  [unwired: 2 in, 2 out]
            n162 = property on="Rev/Fwd" class="Clust (strict)"("Visible"=FALSE) -> ()  [unwired: 2 in, 2 out]
            n163 = case shown="\"White Balance  **\"" w288 {
              tunnel: w287 -> [w294 w303 w312 w321 w330 _ w336]
              tunnel: w286 -> [w292 w300 w309 w318 w327 _ _]
              frame "Size  **" {
                n164 = Index Array(array=w292) -> (element=w291:cluster{string[]})  [unwired: 1 in]
                n165 = call <vilib>:"NT Read String.vi"("Name"=w294) -> ("String"=w293:string)  [unwired: 9 in, 1 out]
                n166 = Unbundle(w291) -> (w289:string[])
                n167 = Match First String(2:w289, 3:w293) -> (0:w290:i32)  [unwired: 1 out]
                n168 = property on="Test Ring" class="Ring (strict)"("Value"=w290, "Strings []"=w289) -> ()  [unwired: 2 in, 2 out]
                n169 = property on="Test Ring" class="Ring (strict)"("Visible"=TRUE) -> ()  [unwired: 2 in, 2 out]
                n170 = property on="Test Slider" class="Slide (strict)"("Visible"=FALSE) -> ()  [unwired: 2 in, 2 out]
              }
              frame "White Balance  **" {
                n171 = Index Array(array=w300, index=1) -> (element=w301:cluster{string[]})
                n172 = call <vilib>:"NT Read String.vi"("Name"=w303) -> ("String"=w302:string)  [unwired: 9 in, 1 out]
                n173 = Unbundle(w301) -> (w298:string[])
                n174 = Match First String(2:w298, 3:w302) -> (0:w297:i32)  [unwired: 1 out]
                n175 = property on="Test Ring" class="Ring (strict)"("Value"=w297, "Strings []"=w298) -> ()  [unwired: 2 in, 2 out]
                n176 = property on="Test Ring" class="Ring (strict)"("Visible"=TRUE) -> ()  [unwired: 2 in, 2 out]
                n177 = property on="Test Slider" class="Slide (strict)"("Visible"=FALSE) -> ()  [unwired: 2 in, 2 out]
              }
              frame "Exposure  **" {
                n178 = Index Array(array=w309, index=2) -> (element=w310:cluster{string[]})
                n179 = call <vilib>:"NT Read String.vi"("Name"=w312) -> ("String"=w311:string)  [unwired: 9 in, 1 out]
                n180 = Unbundle(w310) -> (w306:string[])
                n181 = Match First String(2:w306, 3:w311) -> (0:w307:i32)  [unwired: 1 out]
                n182 = property on="Test Ring" class="Ring (strict)"("Value"=w307, "Strings []"=w306) -> ()  [unwired: 2 in, 2 out]
                n183 = property on="Test Ring" class="Ring (strict)"("Visible"=TRUE) -> ()  [unwired: 2 in, 2 out]
                n184 = property on="Test Slider" class="Slide (strict)"("Visible"=FALSE) -> ()  [unwired: 2 in, 2 out]
              }
              frame "Exposure Priority  **" {
                n185 = Index Array(array=w318, index=3) -> (element=w319:cluster{string[]})
                n186 = call <vilib>:"NT Read String.vi"("Name"=w321) -> ("String"=w320:string)  [unwired: 9 in, 1 out]
                n187 = Unbundle(w319) -> (w315:string[])
                n188 = Match First String(2:w315, 3:w320) -> (0:w316:i32)  [unwired: 1 out]
                n189 = property on="Test Ring" class="Ring (strict)"("Value"=w316, "Strings []"=w315) -> ()  [unwired: 2 in, 2 out]
                n190 = property on="Test Ring" class="Ring (strict)"("Visible"=TRUE) -> ()  [unwired: 2 in, 2 out]
                n191 = property on="Test Slider" class="Slide (strict)"("Visible"=FALSE) -> ()  [unwired: 2 in, 2 out]
              }
              frame "Color Enable  **" {
                n192 = Index Array(array=w327, index=4) -> (element=w328:cluster{string[]})
                n193 = call <vilib>:"NT Read String.vi"("Name"=w330) -> ("String"=w329:string)  [unwired: 9 in, 1 out]
                n194 = Unbundle(w328) -> (w324:string[])
                n195 = Match First String(2:w324, 3:w329) -> (0:w325:i32)  [unwired: 1 out]
                n196 = property on="Test Ring" class="Ring (strict)"("Value"=w325, "Strings []"=w324) -> ()  [unwired: 2 in, 2 out]
                n197 = property on="Test Ring" class="Ring (strict)"("Visible"=TRUE) -> ()  [unwired: 2 in, 2 out]
                n198 = property on="Test Slider" class="Slide (strict)"("Visible"=FALSE) -> ()  [unwired: 2 in, 2 out]
              }
              frame Default {
                n199 = property on="Test Ring" class="Ring (strict)"("Visible"=FALSE) -> ()  [unwired: 2 in, 2 out]
                n200 = property on="Test Slider" class="Slide (strict)"("Visible"=FALSE) -> ()  [unwired: 2 in, 2 out]
              }
              frame "Brightness  **", "Color Level  **", "Compression  **", "FPS  **", "Sharpness  **" {
                n201 = call <vilib>:"NT Read Number.vi"("Name"=w336) -> ("Numeric"=w335:dbl)  [unwired: 9 in, 1 out]
                n202 = local write "Test Slider"(w335) -> ()
                n203 = property on="Test Slider" class="Slide (strict)"("Visible"=TRUE, "Scale.Maximum"=100.0 ("Scale.Range:Maximum")) -> ()  [unwired: 2 in, 2 out]
                n204 = property on="Test Ring" class="Ring (strict)"("Visible"=FALSE) -> ()  [unwired: 2 in, 2 out]
              }
            }
          }
        }
        n205 = property on="Progress" class="Clust (strict)"("Visible"=FALSE) -> ()  [unwired: 2 in, 2 out]
      }
      event "Test Name": Mouse Enter {
        # "Populate the ring with the list of tests"
        n206 = event-data() -> ()  [unwired: 1 in, 1 out]
        n207 = call <vilib>:"NT Read String Array.vi"("Name"="TestMode/TestList") -> ("String Array"=w344:string[])  [unwired: 9 in, 1 out]
        n208 = Build Array (concatenate)("Select the test to run...", w344) -> (w343:string[])
        n209 = property on="Test Name" class="Ring (strict)"("Strings []"=w343) -> ()  [unwired: 2 in, 2 out]
      }
      event "Test Name": Value Change {
        w346 = FALSE ("Visible")
        # "Tell the robot the test name to run"
        n210 = event-data() -> ("NewVal"=w350:u16)  [unwired: 1 in]
        n211 = property on="Test Name" class="Ring (strict)"() -> ("Strings []"=w351:string[])  [unwired: 2 in, 2 out]
        n212 = local write "Progress"(T7 {"Test Progress"=0, "Test Progress Text"=""} ("Progress")) -> ()
        n213 = Index Array(array=w351, index=w350) -> (element=w349:string)
        n214 = call <vilib>:"NT Write String.vi"("String"=w349, "Name"="TestMode/TestName") -> ()  [unwired: 9 in, 1 out]
        n215 = property on="Progress" class="Clust (strict)"("Visible"=TRUE) -> ()  [unwired: 2 in, 2 out]
        n216 = property on="Motor" class="Clust (strict)"("Visible"=w346) -> ()  [unwired: 2 in, 2 out]
        n217 = property on="Test Slider" class="Slide (strict)"("Visible"=w346) -> ()  [unwired: 2 in, 2 out]
        n218 = property on="On/Off" class="Bool (strict)"("Visible"=w346) -> ()  [unwired: 2 in, 2 out]
        n219 = property on="Rev/Fwd" class="Clust (strict)"("Visible"=w346) -> ()  [unwired: 2 in, 2 out]
        n220 = property on="Test Ring" class="Ring (strict)"("Visible"=w346) -> ()  [unwired: 2 in, 2 out]
      }
      event "Listbox": Double Click {
        n221 = event-data() -> ("PlatMods.Shift"=w354:bool, "Row"=w356:i32)  [unwired: 1 in]
        n222 = case shown="True" w354 {
          tunnel: w356 -> [w360 _]
          tunnel: 1 -> [w359 _]
          frame False {
            n223 = property on="Listbox" class="LstBox (strict)"() -> ("Item Symbols"=w358:i32[])  [unwired: 2 in, 2 out]
            n224 = Replace Array Subset(array=w358, new element=w359, index=w360) -> (w357:i32[])
            n225 = property on="Listbox" class="LstBox (strict)"("Item Symbols"=w357) -> ()  [unwired: 2 in, 2 out]
          }
          frame True {
            w361 = 0 ("Top Row")
            n226 = property on="Listbox" class="LstBox (strict)"() -> ("Number of Rows"=w363:u32)  [unwired: 2 in, 2 out]
            n227 = Initialize Array(0, w363) -> (w362:i32[])
            n228 = property on="Listbox" class="LstBox (strict)"("Top Row"=w361, "Value"=w361, "Item Symbols"=w362) -> ()  [unwired: 2 in, 2 out]
          }
        }
      }
      event "Listbox": Key Down {
        n229 = event-data() -> ("VKey"=w367:T20)  [unwired: 1 in]
        n230 = case shown="\"Left\", \"Right\"" w367 {
          selector: w367 -> [w372 _]
          tunnel: eventvkey."Left" ("VKey") -> [w370 _]
          frame "Left", "Right" {
            n231 = Equal?(x=w370, y=w372) -> (x = y?=w371:bool)
            n232 = Select(t=0, s=w371, f=1) -> (s? t:f=w373:i32)
            n233 = property on="Listbox" class="LstBox (strict)"() -> ("Item Symbols"=w376:i32[])  [unwired: 2 in, 2 out]
            n234 = Replace Array Subset(array=w376, new element=w373, index="Listbox") -> (w375:i32[])
            n235 = property on="Listbox" class="LstBox (strict)"("Item Symbols"=w375) -> ()  [unwired: 2 in, 2 out]
          }
          frame Default {
          }
        }
      }
      event "DB Camera Config": Value Change {
        n236 = event-data() -> ("NewVal"=w380:bool)  [unwired: 1 in]
        n237 = case shown="False" w380 {
          tunnel: w379 -> [w389 _]
          tunnel: [w382 w400] -> w378
          tunnel: w377 -> [w381 w400]
          frame False {
            w396 = "Camera"
            w399 = FALSE ("Visible")
            n238 = local read "Camera Settings"() -> (w388:T2)
            n239 = Index Array(array=w389) -> (element=w392:cluster{string[]})  [unwired: 1 in]
            n240 = Unbundle(w388) -> ("Frame Rate"=w387:i32, "Compression"=w386:i32, "Size"=w390:u16)
            n241 = Unbundle(w392) -> (w391:string[])
            n242 = Index Array(array=w391, index=w390) -> (element=w385:string)
            n243 = call-poly <vilib>:"Write Key.vi"("section"=w396, "value"=w385, "key"="Size", "refnum"=w381) -> ("refnum out"=w398:T16)  [unwired: 2 in, 5 out]
            n244 = call-poly <vilib>:"Write Key.vi"("section"=w396, "value"=w387, "key"="FrameRate", "refnum"=w398) -> ("refnum out"=w397:T16)  [unwired: 1 in, 6 out]
            n245 = property on="Camera Settings" class="Clust (strict)"("Visible"=w399) -> ()  [unwired: 2 in, 2 out]
            n246 = local write "DB Camera Config"(w399) -> ()
            n247 = call-poly <vilib>:"Write Key.vi"("section"=w396, "value"=w386, "key"="Compression", "refnum"=w397) -> ("refnum out"=w383:T16)  [unwired: 1 in, 6 out]
            n248 = call <vilib>:"Close Config Data.vi"("refnum"=w383) -> ("file path"=w384:path)  [unwired: 2 in, 8 out]
            n249 = call <vilib>:"Open Config Data.vi"("configuration file path"=w384) -> ("refnum"=w382:T16)  [unwired: 8 in, 2 out]
          }
          frame True {
            n250 = property on="Camera Settings" class="Clust (strict)"("Visible"=TRUE) -> ()  [unwired: 2 in, 2 out]
          }
        }
      }
      event "Camera Settings": Value Change {
        n251 = event-data() -> ("NewVal"=w413:T2)  [unwired: 1 in]
        n252 = Index Array(array=w409) -> (element=w408:cluster{string[]})  [unwired: 1 in]
        n253 = Unbundle(w413) -> ("Frame Rate"=w404:i32, "Compression"=w403:i32, "Size"=w406:u16)
        n254 = Unbundle(w408) -> (w407:string[])
        n255 = Index Array(array=w407, index=w406) -> (element=w405:string)
        n256 = Format Into String(format string="%s   %dfps   %d%%", w405, w404, w403) -> (resulting string=w410:string)  [unwired: 2 in, 1 out]
        n257 = Build Array(w410) -> (w411:string[])
        n258 = property on="DB Camera Config" class="Bool (strict)"("Strings [4]"=w411) -> ()  [unwired: 2 in, 2 out]
      }
      event "Motor.Enable": Value Change {
        n259 = event-data() -> ("NewVal"=w419:bool)  [unwired: 1 in]
        n260 = Unbundle("Motor") -> ("Value"=w418:dbl)  [unwired: 1 out]
        n261 = Select(t=w418, s=w419, f=0.0) -> (s? t:f=w416:dbl)
        n262 = call <vilib>:"NT Write Number.vi"("Numeric"=w416, "Name"=w415) -> ()  [unwired: 9 in, 1 out]
      }
      event "Test Slider": Value Change {
        n263 = event-data() -> ("NewVal"=w422:dbl)  [unwired: 1 in]
        n264 = call <vilib>:"NT Write Number.vi"("Numeric"=w422, "Name"=w423) -> ()  [unwired: 9 in, 1 out]
      }
      event "On/Off": Value Change {
        n265 = event-data() -> ("NewVal"=w427:bool)  [unwired: 1 in]
        n266 = Boolean To (0,1)(Boolean=w427) -> (0, 1=w426:i16)
        n267 = call <vilib>:"NT Write Number.vi"("Numeric"=w426, "Name"=w425) -> ()  [unwired: 9 in, 1 out]
      }
      event "Rev/Fwd": Value Change {
        n268 = event-data() -> ("NewVal.Forward"=w435:bool, "NewVal.Reverse"=w434:bool)  [unwired: 1 in]
        n269 = Boolean To (0,1)(Boolean=w435) -> (0, 1=w431:i16)
        n270 = Boolean To (0,1)(Boolean=w434) -> (0, 1=w433:i16)
        n271 = Negate(x=w433) -> (-x=w432:i16)
        n272 = Add(x=w431, y=w432) -> (x+y=w430:i16)
        n273 = call <vilib>:"NT Write Number.vi"("Numeric"=w430, "Name"=w429) -> ()  [unwired: 9 in, 1 out]
      }
      event "Test Ring": Value Change {
        n274 = event-data() -> ("NewVal"=w439:u16)  [unwired: 1 in]
        n275 = property on="Test Ring" class="Ring (strict)"() -> ("Strings []"=w440:string[])  [unwired: 2 in, 2 out]
        n276 = Index Array(array=w440, index=w439) -> (element=w438:string)
        n277 = call <vilib>:"NT Write String.vi"("String"=w438, "Name"=w437) -> ()  [unwired: 9 in, 1 out]
      }
      event "Rec Mode": Value Change {
        # "Update globals for recording mode and path to read log from.\nClear when logging and let NetworkTables set path for vision to\nuse."
        n278 = event-data() -> ("NewVal"=w450:enum32{"Stop", "Record", "Playback"})  [unwired: 1 in]
        n279 = global write "WPI_DashboardLogging Global.vi" "Logging Filename"(path "") -> ()
        n280 = case shown="\"Stop\", \"Record\"" w450 {
          tunnel: w449 -> [_ w452 w460]
          tunnel: [_ _ w459] -> w446
          tunnel: [_ _ w458] -> _
          tunnel: w444 -> [_ _ w456]
          tunnel: cluster{i32, i32} {-250, 170} -> [_ _ w455]
          tunnel: [_ _ T21 {"Image Size"=TRUE, "Image Type"=TRUE, "Pixel Value"=TRUE, "ROI Information"=TRUE, "Zoom Factor"=FALSE} ("Image Information Shown:All Elements")] -> w442
          tunnel: [_ _ TRUE ("Zoom Factor")] -> w441
          frame Default {
          }
          frame "Stop", "Record" {
            # "Place Window too"
            n281 = invoke class="VI" method="FP.Close"(reference=w452) -> (reference out=w451:refnum<vi>)  [unwired: 2 in, 2 out]
            n282 = invoke class="VI" method="Abort VI"(reference=w451) -> ()  [unwired: 2 in, 3 out]
          }
          frame "Playback" {
            n283 = call "Open Playback Panel.vi"("Offset"=w455, "DB VI Ref"=w456, "Playback in"=w460) -> ("Playback out"=w457:refnum<vi>)  [unwired: 8 in]
            n284 = register-events(w457) -> (reference out=w459:refnum<event-registration>, error out=w458:errorcluster)  [unwired: 2 in]
          }
        }
        n285 = global write "WPI_DashboardLogging Global.vi" "Recording"(w450) -> ()
        n286 = property on="Camera Image" class="ImageControl"("Image Information Shown"=w442, "Image Information Visible"=w441) -> ()  [unwired: 2 in, 2 out]
        n287 = call <vilib>:"WPI_DashboardNT Log FieldName Cache.vi"("Operation"=enum16{"Lookup/Add", "Index", "Clear"}."Clear") -> ()  [unwired: 8 in, 3 out]
      }
      event Panel Close {
        w461 = enum32{"Stop", "Record", "Playback"}."Stop" ("Rec Mode")
        n288 = event-data() -> ()  [unwired: 1 in, 4 out]
        n289 = local write "Rec Mode"(w461) -> ()
        n290 = global write "WPI_DashboardLogging Global.vi" "Recording"(w461) -> ()
      }
      event Panel Close {
        # "Abort playback window and ourself"
        n291 = event-data() -> ()  [unwired: 1 in, 4 out]
        n292 = invoke class="VI" method="FP.Close"(reference=w466) -> (reference out=w465:refnum<vi>)  [unwired: 2 in, 2 out]
        n293 = invoke class="VI" method="Abort VI"(reference=w465) -> (error out=w464:errorcluster)  [unwired: 2 in, 2 out]
        n294 = invoke class="VI" method="Abort VI"(error in=w464) -> ()  [unwired: 2 in, 3 out]
      }
    }
  }
  n295 = property on="On/Off" class="Bool (strict)"("Visible"=w29) -> ()  [unwired: 2 in, 2 out]
  n296 = property on="Motor" class="Clust (strict)"("Visible"=w29) -> ()  [unwired: 2 in, 2 out]
  n297 = property on="Progress" class="Clust (strict)"("Visible"=w29) -> ()  [unwired: 2 in, 2 out]
  n298 = property on="Test Ring" class="Ring (strict)"("Visible"=w29) -> ()  [unwired: 2 in, 2 out]
  n299 = property on="Rev/Fwd" class="Clust (strict)"("Visible"=w29) -> ()  [unwired: 2 in, 2 out]
  n300 = property on="Camera Settings" class="Clust (strict)"("Visible"=w29) -> ()  [unwired: 2 in, 2 out]
  n301 = local write "DB Camera Config"(w29) -> ()
  n302 = global write "WPI_DashboardLogging Global.vi" "Recording"(w12) -> ()
  n303 = local write "Rec Mode"(w12) -> ()
